vi "ProcessJSONSequencedVariables.vi"(8 "error in (no error)":errorcluster, 10 "JSON Array":string) -> (0 "error out":errorcluster, 1 "JSON Error string":string, 3 "JSON Response String":string)   [LabVIEW 2013]
doc: "Takes an array of variable array and separates them into set to be applied after a SetList run sequence finishes.\n\nFor each sub-array, extracts and valiadates the array of JSON Variables before entering them in the appropriate queue for processing. Generates an appropriate JSON response object."
uses:
  JSONVarSet.ctl
  <vilib>/regexp/Match Regular Expression.xnode
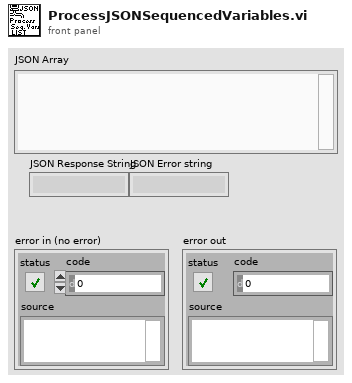
[diagram p1: front panel]
types:
  T1 = typedef "JSONVarSet.ctl" = string[]
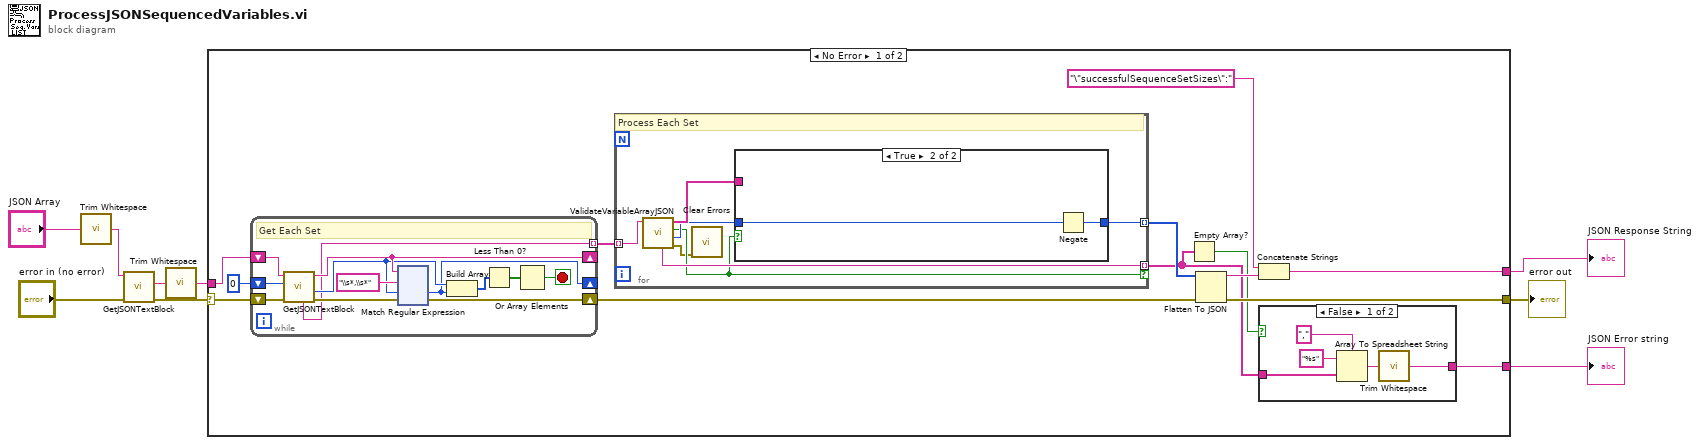
[diagram p0: block diagram]
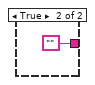
[diagram p2: hidden frame]
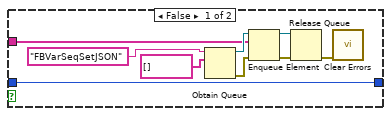
[diagram p3: hidden frame]
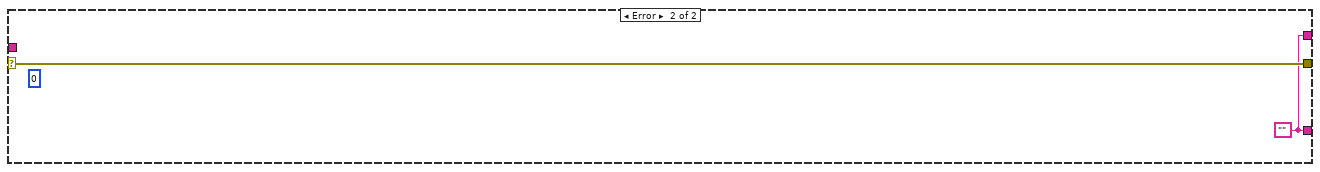
[diagram p4: hidden frame]
diagram:
  n1 = call <vilib>:"Trim Whitespace.vi"("string"="JSON Array") -> ("trimmed string"=w5:string)  [unwired: 1 in]
  n2 = call "GetJSONTextBlock.vi"("error in (no error)"="error in (no error)", "String In"=w5) -> ("error out"=w2:errorcluster, "Matched Block Contents"=w4:string)  [unwired: 5 in, 3 out]
  n3 = call <vilib>:"Trim Whitespace.vi"("string"=w4) -> ("trimmed string"=w1:string)  [unwired: 1 in]
  n4 = case shown="No Error" w2 {
    selector: w2 -> [w10 w175]
    tunnel: w1 -> [w18 _]
    tunnel: [w19 w175] -> w9
    tunnel: [w15 w174] -> w7
    tunnel: [w21 w174] -> w6
    frame No Error {
      n5 = while {
        shift-right: [w49] -> _
        shift-left: 0 ("offset past match") -> [w57]
        shift-right: [w55] -> _
        shift-left: w18 -> [w56]
        shift-right: [w54] -> w12
        shift-left: w10 -> [w53]
        tunnel: [w47] -> w17 mode=indexing
        stop <- w48 stop-if-true
        # "Get Each Set"
        n6 = call "GetJSONTextBlock.vi"("error in (no error)"=w53, "Block Start Offset"=w57, "String In"=w56) -> ("error out"=w58:errorcluster, "Offset Past Block"=w50:i32, "String Out"=w55:string, "Matched Block"=w47:string)  [unwired: 4 in, 1 out]
        n7 = xnode "Match Regular Expression"("input string"=w55, "regular expression"="\\s*,\\s*", "offset (0)"=w50, "error in"=w58) -> ("offset past match"=w49:i32, "error out"=w54:errorcluster)  [unwired: 2 in, 3 out]
        n8 = Build Array(w50, w49) -> (w52:i32[])
        n9 = Less Than 0?(x=w52) -> (x < 0?=w51:bool[])
        n10 = Or Array Elements(Boolean array=w51) -> (logical OR=w48:bool)
      }
      n11 = for {
        tunnel: w17 -> [w35] mode=indexing
        tunnel: [w32] -> w16 mode=indexing
        tunnel: [w31] -> w13 mode=indexing if=w30
        # "Process Each Set"
        n12 = call "ValidateVariableArrayJSON.vi"("JSONVariableArray"=w35) -> ("error out"=w29:errorcluster, "Valid Count"=w33:i32, "InvalidVariables?"=w30:bool, "JSONVarSet"=w34:T1, "JSONErrorResponse"=w31:string)  [unwired: 6 in]
        n13 = call <vilib>:"Clear Errors.vi"("error in (no error)"=w29) -> ()  [unwired: 6 in, 1 out]
        n14 = case shown="True" w30 {
          tunnel: w34 -> [w37 _]
          tunnel: w33 -> [w36 w46]
          tunnel: [w36 w45] -> w32
          frame False {
            n15 = Obtain Queue(name (unnamed)="FBVarSeqSetJSON", element data type=T1 [] ("JSONVarSet")) -> (queue out=w42:refnum<queue>, error out=w43:errorcluster)  [unwired: 3 in, 1 out]
            n16 = Enqueue Element(queue=w42, element=w37, error in (no error)=w43) -> (queue out=w38:refnum<queue>, error out=w39:errorcluster)  [unwired: 1 in, 1 out]
            n17 = Release Queue(queue=w38, error in (no error)=w39) -> (error out=w40:errorcluster)  [unwired: 1 in, 2 out]
            n18 = call <vilib>:"Clear Errors.vi"("error in (no error)"=w40) -> ()  [unwired: 6 in, 1 out]
          }
          frame True {
            n19 = Negate(x=w46) -> (-x=w45:i32)
          }
        }
      }
      n20 = Empty Array?(array=w13) -> (empty?=w14:bool)
      n21 = Flatten To JSON(anything=w16, error in (no error)=w12) -> (JSON string=w20:string, 11:w19:errorcluster)  [unwired: 1 in]
      n22 = Concatenate Strings("\"successfulSequenceSetSizes\":" ("string"), w20) -> (w21:string)
      n23 = case shown="False" w14 {
        tunnel: w13 -> [w25 _]
        tunnel: [w23 ""] -> w15
        frame False {
          n24 = Array To Spreadsheet String(delimiter (Tab)=",", array=w25, 3:"%s" ("format string")) -> (spreadsheet string=w24:string)
          n25 = call <vilib>:"Trim Whitespace.vi"("string"=w24) -> ("trimmed string"=w23:string)  [unwired: 1 in]
        }
        frame True {
        }
      }
    }
    frame Error {
      w174 = ""
      (unwired) 0 ("offset past token")
    }
  }
  "error out" <- w9
  "JSON Error string" <- w7
  "JSON Response String" <- w6
